vi "error log (SubVI).vi"(11 "Enum":T1(ring)) -> (3 "error out 2":errorcluster)   [LabVIEW 2017]
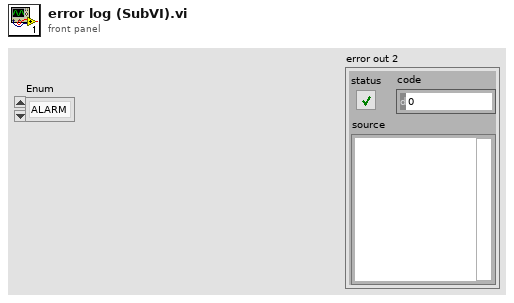
[diagram p1: front panel]
types:
  T1 = enum16{"ALARM", "IZABERI", "CEKAJ", "MERENJE", "POKRENI", "SLIKANJE"}
  T2 = enum16{"open", "replace", "create", "open or create", "replace or create", "replace or create with confirmation"}
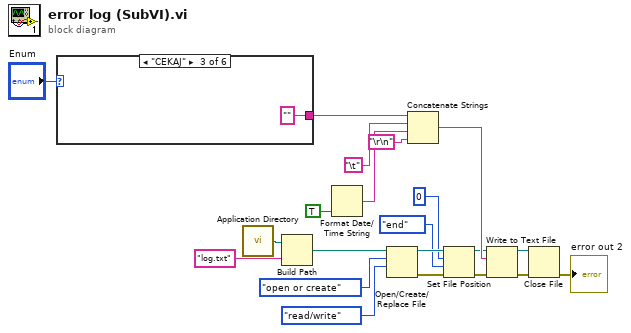
[diagram p0: block diagram]
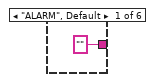
[diagram p2: hidden frame]
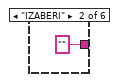
[diagram p3: hidden frame]
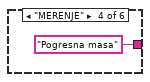
[diagram p4: hidden frame]
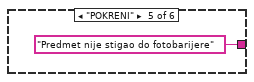
[diagram p5: hidden frame]
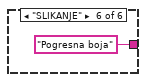
[diagram p6: hidden frame]
diagram:
  n1 = case shown="\"CEKAJ\"" "Enum" {
    tunnel: ["" "" "" "Pogresna masa" "Predmet nije stigao do fotobarijere" "Pogresna boja"] -> w16
    frame "ALARM", Default {
    }
    frame "IZABERI" {
    }
    frame "CEKAJ" {
    }
    frame "MERENJE" {
    }
    frame "POKRENI" {
    }
    frame "SLIKANJE" {
    }
  }
  n2 = call <vilib>:"Application Directory.vi"() -> ("Application Directory"=w7:path)
  n3 = Build Path(base path=w7, name or relative path="log.txt") -> (appended path=w19:path)
  n4 = Format Date/Time String(UTC format=TRUE) -> (date/time string=w14:string)  [unwired: 2 in]
  n5 = Open/Create/Replace File(file path (use dialog)=w19, operation (0:open)=T2."open or create", access (0:read/write)=enum16{"read/write", "read-only", "write-only"}."read/write") -> (refnum out=w6:refnum<file>, error out=w5:errorcluster)  [unwired: 3 in, 1 out]
  n6 = Concatenate Strings(w16, "\t", w14, "\r\n") -> (w11:string)
  n7 = Set File Position(offset (in bytes) (0)=i64 0, refnum=w6, from (0:start)=enum16{"start", "end", "current"}."end", error in=w5) -> (refnum out=w4:refnum<file>, error out=w3:errorcluster)
  n8 = Write to Text File(file (use dialog)=w4, text=w11, error in=w3) -> (refnum out=w9:refnum<file>, error out=w10:errorcluster)  [unwired: 1 in, 1 out]
  n9 = Close File(refnum=w9, error in=w10) -> (error out=→"error out 2":errorcluster)  [unwired: 1 out]
